vi "ZZZ Chroma 1905x Series Get Data.vi"(0 "inst handle in":refnum<visa-resource-name>, 3 "error in":T1) -> (6 "inst handle out":refnum<visa-resource-name>, 7 "Status":string, 9 "error out":T1)   [LabVIEW 2025]
doc: "Chroma\n5 Clock Tower Place Suite 210\nMaynard, MA 01754\nTel: 1 800 253-1230\nTel: 1 877 4 A HIPOT\nFax: 1 978-461-4295\nWebsite: www.chroma.com"
uses:
  <instrlib>/Chroma 19052/Chroma 19052.lvlib
panel:
  out "read buffer":string
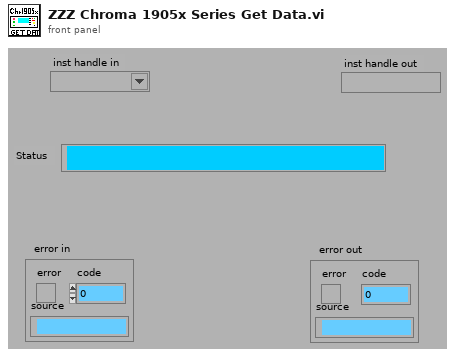
[diagram p1: front panel]
types:
  T1 = cluster{"error":bool, "code":i8, "source":string}
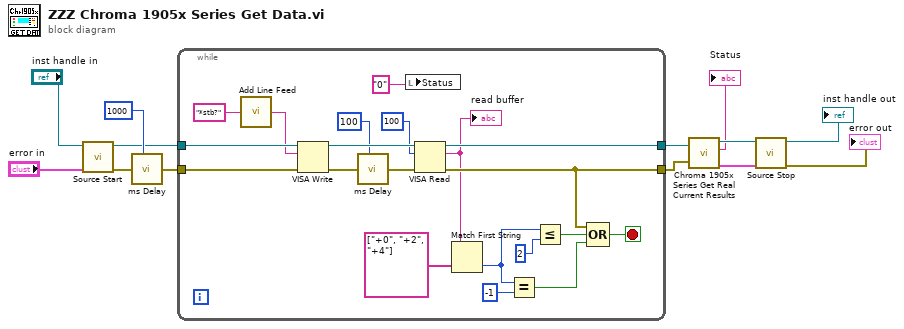
[diagram p0: block diagram]
diagram:
  n1 = call <instrlib>:"Source Start.vi"("error in (no error)"="error in", "VISA resource name"="inst handle in") -> ("error out"=w4:errorcluster, "VISA resource name out"=w1:refnum<visa-resource-name>)  [unwired: 8 in]
  n2 = call <instrlib>:"ms Delay.vi"("miliseconds to wait"=u32 1000 ("Time Delay S"), "error in (no error)"=w4) -> ("error out"=w3:errorcluster)  [unwired: 6 in, 1 out]
  n3 = while {
    tunnel: [w29] -> w12
    tunnel: [w19] -> w13
    tunnel: w1 -> [w31]
    tunnel: w3 -> [w30]
    stop <- w28 stop-if-true
    n4 = call <instrlib>:"Add Line Feed.vi"("Command string"="*stb?") -> ("Concatenated string"=w17:string)  [unwired: 4 in]
    n5 = VISA Write(VISA resource name=w31, write buffer=w17, error in (no error)=w30) -> (VISA resource name out=w33:refnum<visa-resource-name>, error out=w22:errorcluster)  [unwired: 1 out]
    n6 = call <instrlib>:"ms Delay.vi"("miliseconds to wait"=u32 100, "error in (no error)"=w22) -> ("error out"=w21:errorcluster)  [unwired: 6 in, 1 out]
    n7 = local write "Status"("0" ("Status")) -> ()
    n8 = VISA Read(VISA resource name=w33, byte count=100, error in (no error)=w21) -> (VISA resource name out=w29:refnum<visa-resource-name>, read buffer=w16:string, error out=w19:errorcluster)  [unwired: 1 out]
    "read buffer" <- w16
    n9 = Match First String(2:string[] ["+0", "+2", "+4"] ("string array"), 3:w16) -> (0:w24:i32)  [unwired: 1 out]
    n10 = Equal?(x=w24, y=-1) -> (x = y?=w15:bool)
    n11 = Less Or Equal?(x=w24, y=2) -> (x <= y?=w14:bool)
    n12 = Compound Arithmetic op=OR(w19, w14, w15) -> (w28:bool)
  }
  n13 = call "Chroma 1905x Series Get Real Current Results.vi"("inst handle Out"=w12, "error in"=w13) -> ("inst handle in"=w8:refnum<visa-resource-name>, "Result"=→"Status":string, "error out"=w11:T1)  [unwired: 1 in]
  n14 = call <instrlib>:"Source Stop.vi"("error in (no error)"=w11, "VISA resource name"=w8) -> ("error out"=→"error out":errorcluster, "VISA resource name out"=→"inst handle out":refnum<visa-resource-name>)  [unwired: 8 in]
